vi "display_active_track_snippets.vi"(0 "Selected Track Index":i32, 2 "error in":errorcluster) -> (3 "Latest Active Worm Tracks":T1[](array[typedef]), 4 "Active Tracks Count":i32, 5 "Mature Tracks Count":i32, 6 "error out":errorcluster)   [LabVIEW 2019]
uses:
  WormTrackSnippetCluster.ctl
  TrackTerminationReasonEnum.ctl
  ActiveTracksFunctionalGlobalOperations.ctl
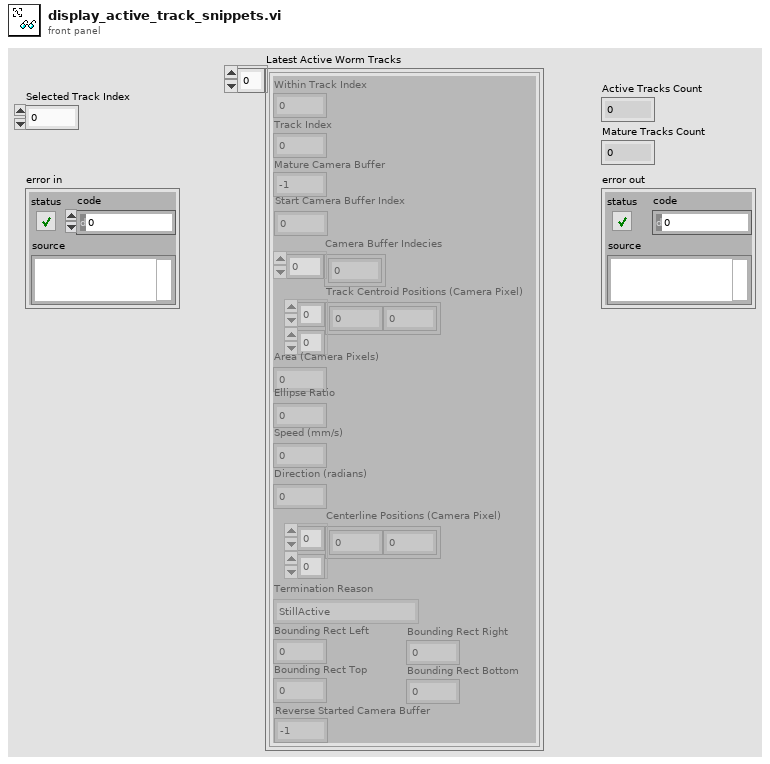
[diagram p1: front panel]
types:
  T1 = typedef "WormTrackSnippetCluster.ctl" = cluster{"Track Centroid Positions (Camera Pixel)":sgl[][], "Within Track Index":i32, "Camera Buffer Indecies":i32[], "Area (Camera Pixels)":i32, "Speed (mm/s)":sgl, "Direction (radians)":sgl, "Centerline Positions (Camera Pixel)":sgl[][], "Ellipse Ratio":sgl, "Termination Reason":T2, "Track Index":i32, "Bounding Rect Left":i32, "Bounding Rect Top":i32, "Bounding Rect Right":i32, "Bounding Rect Bottom":i32, "Mature Camera Buffer":i32, "Start Camera Buffer Index":i32, "Reverse Started Camera Buffer":i32}
  T2 = typedef "TrackTerminationReasonEnum.ctl" = enum16{"StillActive", "MaxDisplacement", "NoBlobsLeft", "AreaIncrease", "AreaDecrease", "ExperimentEnded"}
  T3 = typedef "ActiveTracksFunctionalGlobalOperations.ctl" = enum16{"Initialize", "ReadFullTrackGivenWormIndex", "WriteFullTrack", "ReadTrackSnippets", "WriteTrackGivenSnippets", "ReadStimulusSnippets", "StartNewTracksGivenSnippets", "EndTracksGivenSnippets", "WriteStimulusObjectGivenWormIndex", "CompleteAllActiveTracks", "ReturnAllActiveTrackIndecies"}
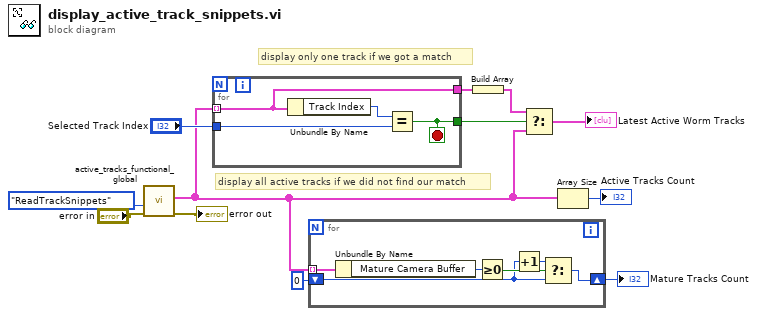
[diagram p0: block diagram]
diagram:
  # "display only one track if we got a match"
  # "display all active tracks if we did not find our match"
  n1 = call "active_tracks_functional_global.vi"("error in"="error in", "Operations"=ActiveTracksFunctionalGlobalOperations."ReadTrackSnippets") -> ("error out"=→"error out":errorcluster, "Track Snippets Out"=w3:T1[])  [unwired: 5 in, 3 out]
  n2 = for {
    tunnel: w3 -> [w14] mode=indexing
    tunnel: [w15] -> w11
    tunnel: [w14] -> w12
    tunnel: "Selected Track Index" -> [w13]
    stop <- w15 stop-if-true
    n3 = Unbundle By Name(w14) -> ("Track Index"=w16:i32)
    n4 = Equal?(x=w16, y=w13) -> (x = y?=w15:bool)
  }
  n5 = for {
    tunnel: w3 -> [w22] mode=indexing
    shift-right: [w19] -> w1
    shift-left: 0 -> [w18]
    n6 = Unbundle By Name(w22) -> ("Mature Camera Buffer"=w21:i32)
    n7 = Greater Or Equal To 0?(x=w21) -> (x >= 0?=w20:bool)
    n8 = Increment(x=w18) -> (x+1=w17:i32)
    n9 = Select(t=w17, s=w20, f=w18) -> (s? t:f=w19:i32)
  }
  "Mature Tracks Count" <- w1
  n10 = Build Array(w12) -> (w10:T1[])
  n11 = Select(t=w10, s=w11, f=w3) -> (s? t:f=→"Latest Active Worm Tracks":T1[])
  n12 = Array Size(array=w3) -> (size(s)=→"Active Tracks Count":i32)
